vi "E710_Scandemo_3D.vi"() -> ()   [LabVIEW 2011]
doc: "This VI demonstrates how to statically define an E-710 configuration with one connected axis. In this example the E-710 is connected through COM port 1 with baudrate 57600. The VI runs E710_Configuration_Setup.vi with these specified settings, performs an automated zero-point calibration of the connected axis and reads the position of the axis. The diagram shows how to combine the driver VIs for these tasks. \n\nWarning: Before running this VI, modify the \"Interface\" and \"RS232 settings\" to reflect your configuration. The predefined settings provided with the VI probably do not match your system."
panel:
  out "ATZ successful?":bool[](array[boolean])
  out "Current Z pane":i32
  out "Referencing":bool
  out "Writing":bool
  out "WG runs":bool
  out "# Wavepoints X/Y":i32=1000
  in  "Startpoint X":dbl format="%.2f"
  in  "stop":bool
  in  "WGO":bool
  in  "WAV":bool
  in  "Trigger every...":dbl=1.0 format="%.2f"
  in  "Stepsize Z":dbl=1.0 min=0.01 step=0.01 format="%.2f"
  in  "Stepsize Y":dbl=5.0 min=0.01 step=0.01 format="%.2f"
  in  "Scanspeed":dbl=1000.0 format="%.2f"
  in  "Startpoint Z":dbl format="%.2f"
  in  "Startpoint Y":dbl format="%.2f"
  in  "Scanrange Z":dbl=10.0 format="%.2f"
  in  "Scanrange Y":dbl=10.0 format="%.2f"
  in  "Scanrange X":dbl=100.0 format="%.2f"
  out "error out":errorcluster
  out "Conn. Axis":string[](array[string])
  out "Identification":string
  # "E-710 3D-Scanning sample"
  # "The unidirectional scan in the XY-pane is based solely on wavegenerator motions.  With SPA the number of wavegenerator\ncycles is limited. After it stops the stage is lifted in the Z-direction and the next scan in the XY-pane is done. Connected\nstages are referenced and autozero'ed first. Scanrange XYZ defines the scanned cuboid. Startpoint XYZ defines its corner\nwhere the scan starts from. Stepsize is the spacing beetween two scanning lines. Trigger output on line 1.\n\nWarning: Before running this VI, modify the \"Interface\" and \"RS232 settings\" to reflect \nyour configuration. The predefined settings probably do not match your system."
  # "Axes are referencing"
  # "µm"
  # "µm"
  # "µm/s"
  # "Writing waveforms"
  # "Wavegen running"
  # "µm"
  # "µm"
  # "µm"
  # "µm"
  # "µm"
  # "µm"
  # "µm"
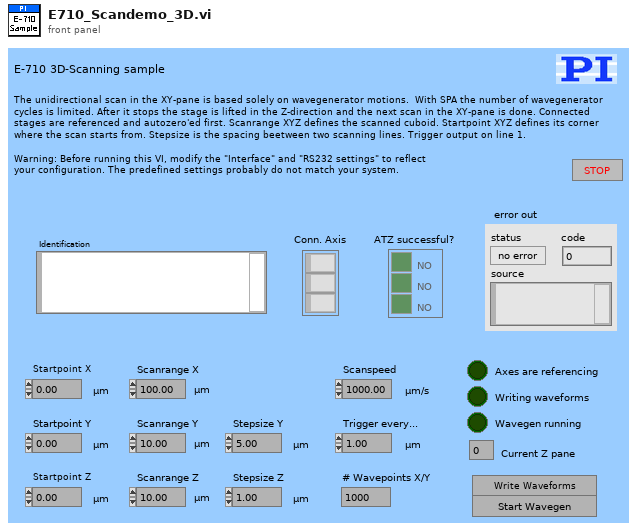
[diagram p1: front panel]
types:
  T1 = cluster{"Conn. Axes[0]":string, "Conn. Axes[1]":string, "Conn. Axes[2]":string}
  T2 = cluster{"PointsX":dbl, "J":dbl, "Scanrange X":dbl, "J":dbl}
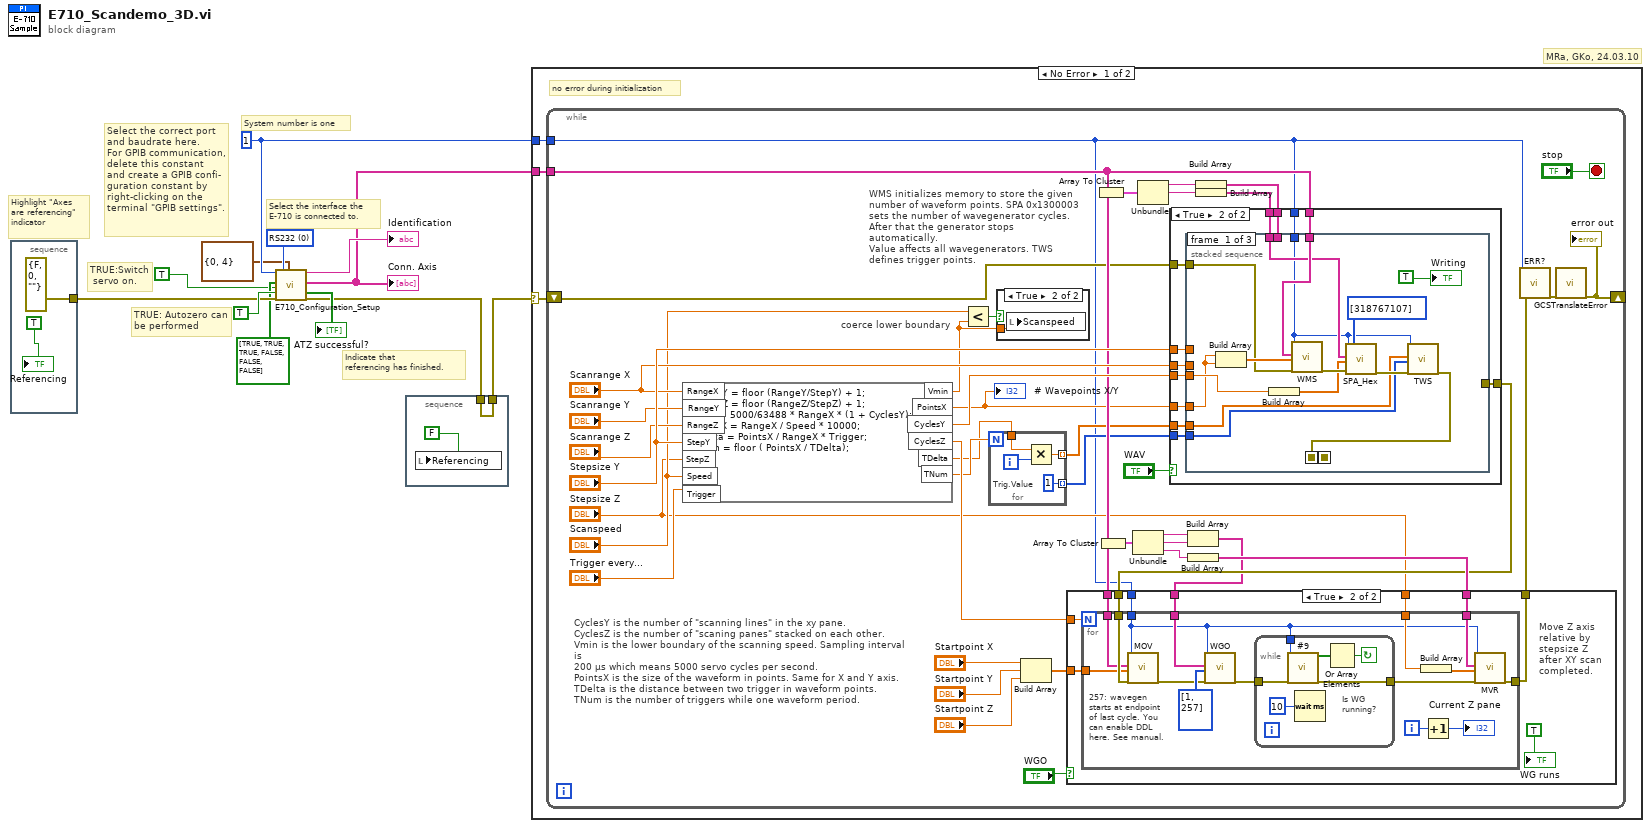
[diagram p0: block diagram]
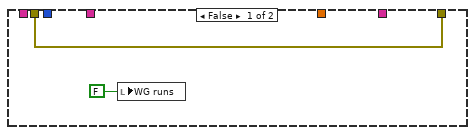
[diagram p2: hidden frame]
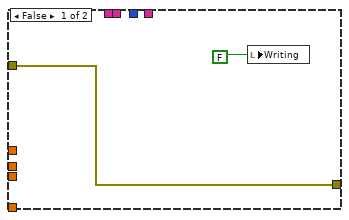
[diagram p4: hidden frame]
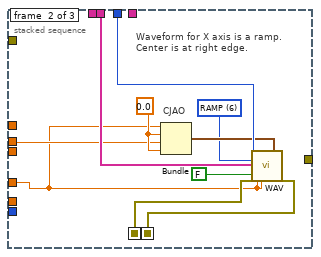
[diagram p5: hidden frame]
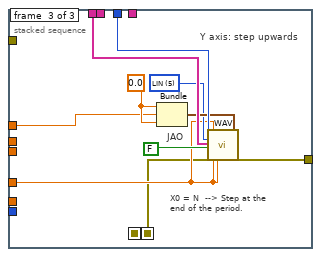
[diagram p6: hidden frame]
diagram:
  w8 = u16 0 items=["RS232", "GPIB"] ("Interface")
  w10 = 1 ("System no.")
  # "TRUE:Switch\n servo on."
  # "Select the interface the\nE-710 is connected to."
  # "Select the correct port \nand baudrate here.\nFor GPIB communication, \ndelete this constant\nand create a GPIB confi-\nguration constant by\nright-clicking on the \nterminal \"GPIB settings\"."
  # "MRa, GKo, 24.03.10"
  # "Indicate that\nreferencing has finished."
  # "Highlight \"Axes\nare referencing\"\nindicator"
  # "TRUE: Autozero can\nbe performed"
  # "System number is one"
  n1 = stacked-sequence {
    tunnel: [errorcluster {"status"=FALSE, "code"=0, "source"=""} ("error out")] -> w9
    frame #0 {
      "Referencing" <- TRUE ("Running")
    }
  }
  n2 = call "E710_Configuration_Setup.vi"("System no."=w10, "Are stages connected?"=bool[] [TRUE, TRUE, TRUE, FALSE, FALSE, FALSE], "Change servo \nstatus to ON?"=TRUE ("Change servo \nstatus to ON?"), "Perform autozero?"=TRUE ("All axes?"), "error in"=w9, "Interface"=w8, "RS232 settings"=cluster{"Portnumber 2":i32, "Baudrate":u16} {"Portnumber 2"=0, "Baudrate"=4}) -> ("Identification"=→"Identification":string, "Conn. Axes"=w4:string[], "ATZ successful?"=→"ATZ successful?":bool[], "error out"=w1:errorcluster)  [unwired: 5 in, 4 out]
  "Conn. Axis" <- w4
  n3 = stacked-sequence {
    tunnel: w1 -> [w15]
    tunnel: [w15] -> w2
    frame #0 {
      n4 = local write "Referencing"(FALSE ("Running")) -> ()
    }
  }
  n5 = case shown="No Error" w2 {
    selector: w2 -> [w17 _]
    tunnel: w10 -> [w19 _]
    tunnel: w4 -> [w18 _]
    frame No Error {
      # "no error during initialization"
      n6 = while {
        shift-left: w17 -> [w25]
        shift-right: [w23] -> _
        tunnel: w18 -> [w34]
        tunnel: w19 -> [w20]
        stop <- "stop" stop-if-true
        # "coerce lower boundary"
        # "WMS initializes memory to store the given\nnumber of waveform points. SPA 0x1300003\nsets the number of wavegenerator cycles. \nAfter that the generator stops automatically.\nValue affects all wavegenerators. TWS\ndefines trigger points."
        # "CyclesY is the number of \"scanning lines\" in the xy pane.\nCyclesZ is the number of \"scaning panes\" stacked on each other.\nVmin is the lower boundary of the scanning speed. Sampling interval is\n200 µs which means 5000 servo cycles per second.\nPointsX is the size of the waveform in points. Same for X and Y axis.\nTDelta is the distance between two trigger in waveform points.\nTNum is the number of triggers while one waveform period."
        n7 = formula code="CyclesY = floor (RangeY/StepY) + 1;\nCyclesZ = floor (RangeZ/StepZ) + 1;\nVmin = 5000/63488 * RangeX * (1 + CyclesY);\nPointsX = RangeX / Speed * 10000;\nTDelta = PointsX / RangeX * Trigger;\nTNum = floor ( PointsX / TDelta);"("RangeX"="Scanrange X", "RangeY"="Scanrange Y", "RangeZ"="Scanrange Z", "StepY"="Stepsize Y", "StepZ"="Stepsize Z", "Speed"="Scanspeed", "Trigger"="Trigger every...") -> ("Vmin"=w29:dbl, "CyclesY"=w50:dbl, "CyclesZ"=w47:dbl, "PointsX"=w32:dbl, "TDelta"=w28:dbl, "TNum"=w31:dbl)
        "# Wavepoints X/Y" <- w32
        n8 = Less?(x="Scanspeed", y=w29) -> (x < y?=w55:bool)
        n9 = for {
          N: w31 -> [_]
          tunnel: w28 -> [w64]
          tunnel: [w62] -> w27 mode=indexing
          tunnel: [1] -> w26 mode=indexing
          i -> [w63]
          # "Trig.Value"
          n10 = Multiply(x=w64, y=w63) -> (x*y=w62:dbl)
        }
        n11 = case shown="True" w55 {
          tunnel: w29 -> [_ w98]
          frame False {
          }
          frame True {
            n12 = local write "Scanspeed"(w98) -> ()
          }
        }
        n13 = Build Array("Startpoint X", "Startpoint Y", "Startpoint Z") -> (w38:dbl[])
        n14 = Array To Cluster(array=w34) -> (cluster=w37:T1)
        n15 = Array To Cluster(array=w34) -> (cluster=w44:T1)
        n16 = Unbundle(w44) -> ("Conn. Axes[0]"=w43:string, "Conn. Axes[1]"=w42:string, "Conn. Axes[2]"=w41:string)
        n17 = Unbundle(w37) -> ("Conn. Axes[0]"=w46:string, "Conn. Axes[1]"=w45:string)  [unwired: 1 out]
        n18 = Build Array(w43, w42) -> (w22:string[])
        n19 = Build Array(w41) -> (w40:string[])
        n20 = Build Array(w46) -> (w59:string[])
        n21 = Build Array(w45) -> (w58:string[])
        n22 = case shown="True" "WAV" {
          tunnel: w20 -> [_ w113]
          tunnel: w59 -> [_ w112]
          tunnel: w34 -> [_ w111]
          tunnel: w58 -> [_ w108]
          tunnel: w32 -> [_ w110]
          tunnel: w50 -> [_ w109]
          tunnel: "Stepsize Y" -> [_ w107]
          tunnel: "Scanrange X" -> [_ w106]
          tunnel: [w99 w105] -> w36
          tunnel: w27 -> [_ w104]
          tunnel: w26 -> [_ w103]
          tunnel: w25 -> [w99 w102]
          frame False {
            n23 = Number To Boolean Array(number=0) -> ()  [unwired: 1 out]
            n24 = local write "Writing"(FALSE) -> ()
          }
          frame True {
            n25 = stacked-sequence {
              seq-local: [w118 _ _] -> [_ w130 _]
              seq-local: [_ w135 _] -> [_ _ w139]
              tunnel: w113 -> [w115 w138 w148]
              tunnel: w112 -> [_ w136 _]
              tunnel: w111 -> [w125 _ _]
              tunnel: w110 -> [w121 w129 w143]
              tunnel: w109 -> [w123 _ _]
              tunnel: w108 -> [w124 _ w147]
              tunnel: w107 -> [_ _ w141]
              tunnel: w106 -> [_ w131 _]
              tunnel: [_ _ w140] -> w105
              tunnel: w104 -> [w117 _ _]
              tunnel: w103 -> [w116 _ _]
              tunnel: w102 -> [w114 _ _]
              frame #0 {
                n26 = Build Array(w121, w121) -> (w128:dbl[])
                n27 = Build Array(w123) -> (w122:dbl[])
                n28 = call "WMS.vi"("System no."=w115, "Axes to set"=w125, "Wave storage max."=w128, "error in"=w114) -> ("error out"=w126:errorcluster)  [unwired: 1 in, 14 out]
                n29 = call "SPA_Hex.vi"("System no."=w115, "Designator to set"=w124, "Parameter value"=w122, "error in"=w126, "Parameter number (hex)"=u32[] [318767107]) -> ("error out"=w119:errorcluster)  [unwired: 1 in, 13 out]
                n30 = call "TWS.vi"("System no."=w115, "Wavepoint"=w117, "Trigger value"=w116, "error in"=w119) -> ("error out"=w118:errorcluster)  [unwired: 1 in, 14 out]
                "Writing" <- TRUE
              }
              frame #1 {
                w132 = u16 6 items=["SIN", "POL", "TAN", "PNT", "SIN_P", "LIN", "RAMP"] ("Waveform")
                w133 = 0.0 ("J")
                # "Waveform for X axis is a ramp.\nCenter is at right edge."
                # "CJAO"
                n31 = Bundle("PointsX"=w129, "J"=w133, "Scanrange X"=w131, "J"=w133) -> (w134:T2)  [unwired: 1 out]
                n32 = call "WAV.vi"("System no."=w138, "Waveform"=w132, "Affected axes"=w136, "Append? (&)"=FALSE, "error in"=w130, "N"=w129, "Segment length"=w129, "RAMP Parameters"=w134) -> ("error out"=w135:errorcluster)  [unwired: 10 in, 9 out]
              }
              frame #2 {
                w145 = u16 5 items=["SIN", "POL", "TAN", "PNT", "SIN_P", "LIN", "RAMP"] ("Waveform")
                w142 = 0.0 ("J")
                # "Y axis: step upwards"
                # "X0 = N  --> Step at the\nend of the period."
                # "JAO"
                n33 = Bundle("J"=w142, "Stepsize Y"=w141, "J"=w142) -> (w146:cluster{"J":dbl, "Stepsize Y":dbl, "J":dbl})  [unwired: 1 out]
                n34 = call "WAV.vi"("System no."=w148, "Waveform"=w145, "Affected axes"=w147, "Append? (&)"=FALSE, "error in"=w139, "Xo"=w143, "N"=w143, "Segment length"=w143, "LIN Parameters"=w146) -> ("error out"=w140:errorcluster)  [unwired: 9 in, 9 out]
              }
            }
          }
        }
        n35 = case shown="True" "WGO" {
          tunnel: w47 -> [_ w76]
          tunnel: w36 -> [w65 w75]
          tunnel: "Stepsize Z" -> [_ w74]
          tunnel: w40 -> [_ w72]
          tunnel: w22 -> [_ w71]
          tunnel: w38 -> [_ w70]
          tunnel: w34 -> [_ w69]
          tunnel: w20 -> [_ w68]
          tunnel: [w65 w67] -> w21
          frame False {
            n36 = local write "WG runs"(FALSE) -> ()
          }
          frame True {
            # "Move Z axis\nrelative by\nstepsize Z\nafter XY scan\ncompleted."
            n37 = for {
              N: w76 -> [_]
              tunnel: [w87] -> w67
              tunnel: w75 -> [w81]
              tunnel: w74 -> [w85]
              tunnel: w72 -> [w83]
              tunnel: w71 -> [w86]
              tunnel: w70 -> [w80]
              tunnel: w69 -> [w79]
              tunnel: w68 -> [w77]
              i -> [w88]
              # "257: wavegen\nstarts at endpoint\nof last cycle. You\ncan enable DDL\nhere. See manual."
              n38 = call "MOV.vi"("System no."=w77, "Axes to move"=w79, "Position values"=w80, "error in"=w81) -> ("error out"=w82:errorcluster)  [unwired: 1 in, 14 out]
              n39 = call "WGO.vi"("System no."=w77, "Affected axes"=w86, "WGO Parameter"=i32[] [1, 257], "error in"=w82) -> ("error out"=w90:errorcluster)  [unwired: 15 out]
              n40 = while {
                tunnel: w77 -> [w92]
                tunnel: [w93] -> w89
                tunnel: w90 -> [w97]
                stop <- w95 continue-if-true
                # "Is WG\nrunning?"
                n41 = call "#9.vi"("System no."=w92, "error in"=w97) -> ("WG running?"=w96:bool[], "error out"=w93:errorcluster)  [unwired: 16 out]
                n42 = Wait (ms)(milliseconds to wait=u32 10) -> ()  [unwired: 1 out]
                n43 = Or Array Elements(Boolean array=w96) -> (logical OR=w95:bool)
              }
              n44 = Build Array(w85) -> (w84:dbl[])
              n45 = Increment(x=w88) -> (x+1=→"Current Z pane":i32)
              n46 = call "MVR.vi"("System no."=w77, "Axes to move"=w83, "Position values"=w84, "error in"=w89) -> ("error out"=w87:errorcluster)  [unwired: 1 in, 14 out]
            }
            "WG runs" <- TRUE
          }
        }
        n47 = call "ERR?.vi"("System no."=w20, "error in"=w21) -> ("error out"=w54:errorcluster)  [unwired: 17 out]
        n48 = call "GCSTranslateError.vi"("error in"=w54) -> ("error out"=w23:errorcluster)  [unwired: 18 out]
        "error out" <- w23
      }
    }
    frame Error {
      # "Error during initialization,\nstop execution here."
    }
  }
